vi "SV TDMS Write Position Info.vi"(0 "tdms file":refnum<k34>, 5 "group name in":string, 7 "channel name in":string, 9 "speed position info":T1, 11 "error in (no error)":errorcluster) -> (4 "tdms file out":refnum<k34>, 6 "group name out":string, 8 "channel name out":string, 15 "error out":errorcluster)   [LabVIEW 2017]
uses:
  <vilib>/addons/_NISVFA/_Shared subVIs/Controls/svc_Position Info.ctl
  <vilib>/addons/_NISVFA/_Shared subVIs/Controls/SV Channel Properties.ctl
  <vilib>/addons/_NISVFA/_Shared subVIs/Controls/NI Channel Properties.ctl
  <vilib>/addons/_NISVFA/_Shared subVIs/Controls/LV Datatypes.ctl
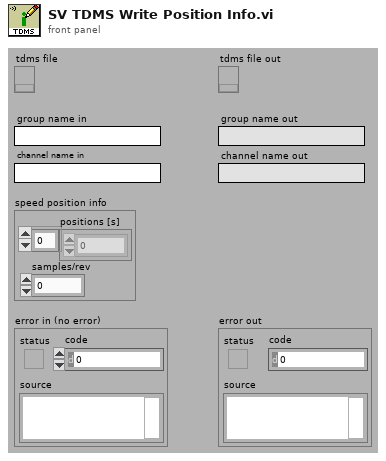
[diagram p1: front panel]
types:
  T1 = typedef "svc_Position Info.ctl" = cluster{"positions [s]":dbl[], "samples/rev":dbl}
  T2 = typedef "LV Datatypes.ctl" = i32
  T3 = typedef "NI Channel Properties.ctl" = u16
  T4 = typedef "SV Channel Properties.ctl" = u16
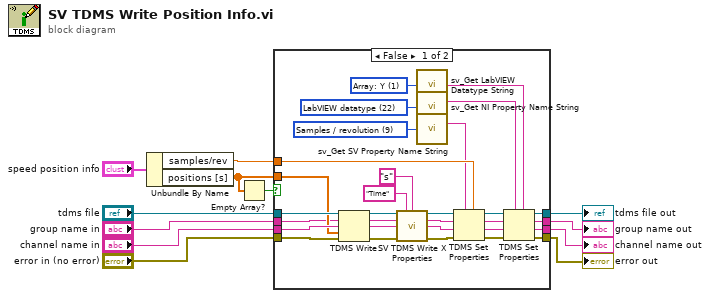
[diagram p0: block diagram]
diagram:
  n1 = Unbundle By Name("speed position info") -> ("samples/rev"=w12:dbl, "positions [s]"=w2:dbl[])
  n2 = Empty Array?(array=w2) -> (empty?=w1:bool)
  n3 = case shown="False" w1 {
    tunnel: w12 -> [w42 _]
    tunnel: "error in (no error)" -> [w41 w43]
    tunnel: "channel name in" -> [w40 w44]
    tunnel: "tdms file" -> [w39 w46]
    tunnel: w2 -> [w38 _]
    tunnel: "group name in" -> [w37 w45]
    tunnel: [w28 w43] -> w6
    tunnel: [w27 w44] -> w5
    tunnel: [w26 w45] -> w4
    tunnel: [w25 w46] -> w3
    frame False {
      w34 = T2 1 items=["String: abc"=-2, "Boolean: True or False"=-1, "Scalar: y"=0, "Array: Y"=1, "Waveform: t0, dt, Y, variant"=2, "Cluster: x0, dx, Y"=3, "Cluster: X, Y"=4, "Waterfall"=5, "Colormap"=6] ("LabVIEW datatype")
      w33 = T3 22 items=["Channel name", "Channel description", "Y-axis label", "Y-axis unit string", "X-axis label", "X-axis unit string", "x0", "dx", "Number of samples", "X channel", "Filter settled", "dB reference", "Window", "Window parameter", "Window size", "FFT size", "Peak units", "Spectrum type", "Magnitude scale", "Spectral density", "Sensor sensitivity (mV/EU)", "X-axis domain", "LabVIEW datatype"] ("property")
      w36 = T4 9 items=["Engineering units", "Custom unit label", "Weighting filter", "Pregain", "Octave standard", "Octave bandwidth", "Octave low band", "Octave high band", "Spectrum skewed", "Samples / revolution"] ("SV property")
      n4 = TDMS Write(0:w39, 5:w37, 7:w40, 9:w38, 11:w41) -> (4:w20:refnum<k34>, 6:w21:string, 8:w17:string, 15:w22:errorcluster)  [unwired: 1 in]
      n5 = call <vilib>:"SV TDMS Write X Properties.vi"("tdms file in"=w20, "X-axis label"="Time", "X-unit string"="s", "group name"=w21, "channel name"=w17, "error in"=w22) -> ("tdms file out"=w19:refnum<k34>, "group name"=w18:string, "channel name"=w16:string, "error out"=w15:errorcluster)  [unwired: 6 in]
      n6 = call <vilib>:"sv_Get LabVIEW Datatype String.vi"("LabVIEW datatype"=w34) -> ("datatype string"=w23:string)  [unwired: 4 in]
      n7 = call <vilib>:"sv_Get NI Property Name String.vi"("property"=w33) -> ("TDMS property name"=w24:string)  [unwired: 13 in, 1 out]
      n8 = call <vilib>:"sv_Get SV Property Name String.vi"("property"=w36) -> ("TDMS property name"=w35:string)  [unwired: 13 in, 1 out]
      n9 = TDMS Set Properties(5:w42, 7:w35, 8:w15, 9:w16, 10:w18, 11:w19) -> (0:w32:errorcluster, 1:w31:string, 2:w30:string, 3:w29:refnum<k34>)
      n10 = TDMS Set Properties(5:w23, 7:w24, 8:w32, 9:w31, 10:w30, 11:w29) -> (0:w28:errorcluster, 1:w27:string, 2:w26:string, 3:w25:refnum<k34>)
    }
    frame True {
    }
  }
  "error out" <- w6
  "channel name out" <- w5
  "group name out" <- w4
  "tdms file out" <- w3
